vi "RS_FSP_SAve to datafile (SubVI).vi"(8 "Error In":errorcluster, 10 "Driver Name":T1, 11 "output":string) -> (0 "error out":errorcluster)   [LabVIEW 2018]
uses:
  MOKO_LabViewLibrary/MokoLowLevel/MokoLowLovelControl/MLLC_DriverName.ctl
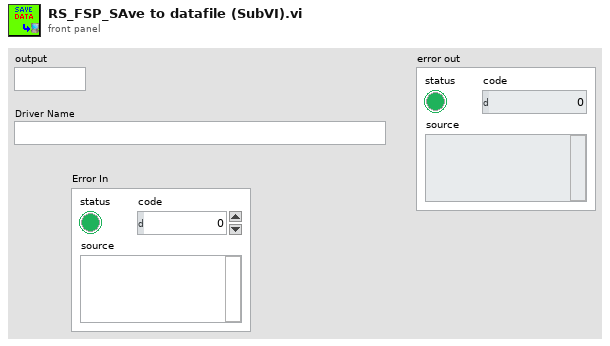
[diagram p1: front panel]
types:
  T1 = typedef "MLLC_DriverName.ctl" = string
  T2 = enum16{"open", "replace", "create", "open or create", "replace or create", "replace or create with confirmation"}
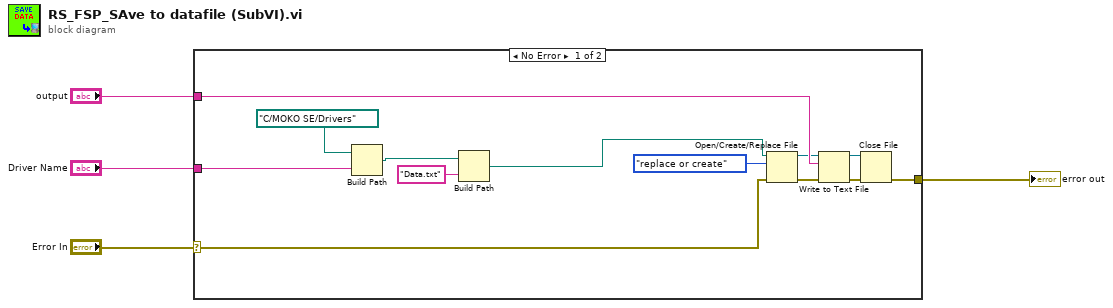
[diagram p0: block diagram]
diagram:
  n1 = case shown="No Error" "Error In" {
    selector: "Error In" -> [w5 w18]
    tunnel: "output" -> [w16 _]
    tunnel: [w15 w18] -> w3
    tunnel: "Driver Name" -> [w8 _]
    frame No Error {
      n2 = Build Path(base path=path "C:/MOKO SE/Drivers" ("directory path"), name or relative path=w8) -> (appended path=w7:path)
      n3 = Build Path(base path=w7, name or relative path="Data.txt") -> (appended path=w10:path)
      n4 = Open/Create/Replace File(file path (use dialog)=w10, error in=w5, operation (0:open)=T2."replace or create") -> (refnum out=w12:refnum<file>, error out=w11:errorcluster)  [unwired: 3 in, 1 out]
      n5 = Write to Text File(file (use dialog)=w12, text=w16, error in=w11) -> (refnum out=w13:refnum<file>, error out=w14:errorcluster)  [unwired: 1 in, 1 out]
      n6 = Close File(refnum=w13, error in=w14) -> (error out=w15:errorcluster)  [unwired: 1 out]
    }
    frame Error {
    }
  }
  "error out" <- w3
